vi "Relay Control - Set Property.vi"(7 "relay action (Close Relay)":T1=enum."Close Relay", 8 "error in (no error)":errorcluster, 10 "Property":refnum<k21>, 11 "SLSC Switch in":refnum<class "SLSC Switch.lvclass">) -> (0 "error out":errorcluster, 3 "SLSC Switch out":refnum<class "SLSC Switch.lvclass">)   [LabVIEW 2015, in "SLSC Switch.lvclass"]
uses:
  SLSC Switch.lvclass
  slscsl/RelayAction.ctl
  SLSC Switch.lvclass/SLSC Switch.ctl
  <vilib>/SLSC/Set Device Property (Bool).vi
  <vilib>/SLSC/Commit Properties for Devices.vi
  <vilib>/SLSC/SLSC.lvlib
  slscsl/slscsl.lvclass
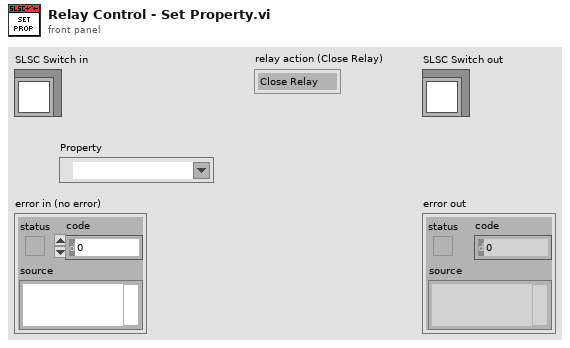
[diagram p1: front panel]
types:
  T1 = typedef "slscsl.lvclass/RelayAction.ctl" = enum16{"Open Relay", "Close Relay"}
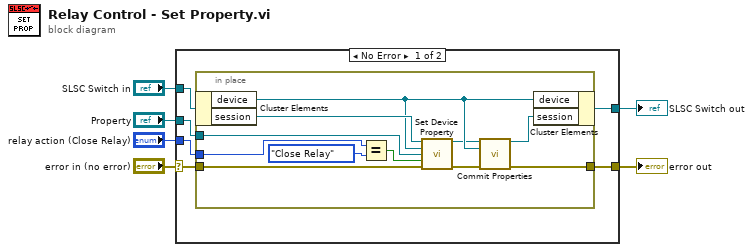
[diagram p0: block diagram]
diagram:
  n1 = case shown="No Error" "error in (no error)" {
    selector: "error in (no error)" -> [w7 w25]
    tunnel: [w11 w25] -> w5
    tunnel: [w10 w24] -> w3
    tunnel: "SLSC Switch in" -> [w9 w24]
    tunnel: "relay action (Close Relay)" -> [w12 _]
    tunnel: "Property" -> [w8 _]
    frame No Error {
      n2 = in-place {
        in-place-border: w12 -> [w17]
        in-place-border: [w22] -> w11
        in-place-border: w7 -> [w21]
        in-place-border: w8 -> [w18]
        n3 = in-place-cluster #1(w9) -> ("device"=w19:refnum<k21>, "session"=w20:refnum<k21>)
        n4 = Equal?(x=w17, y=RelayAction."Close Relay") -> (x = y?=w15:bool)
        n5 = call-poly <vilib>:"Set Device Property.vi"("session in"=w20, "devices"=w19, "property"=w18, "property value"=w15, "error in (no error)"=w21) -> ("session out"=w14:refnum<k21>, "error out"=w13:errorcluster)  [unwired: 9 in]
        n6 = call-poly <vilib>:"Commit Properties.vi"("session in"=w14, "devices"=w19, "error in (no error)"=w13) -> ("session out"=w23:refnum<k21>, "error out"=w22:errorcluster)  [unwired: 11 in]
        n7 = in-place-cluster #1("device"=w19, "session"=w23) -> (w10:refnum<class "SLSC Switch.lvclass">)
      }
    }
    frame Error {
    }
  }
  "error out" <- w5
  "SLSC Switch out" <- w3
